vi "Select Display Mode.vi"(8 "error in (no error)":errorcluster, 10 "DisplayMode":T1, 11 "Instruments in":refnum<class "Instruments.lvclass">) -> (0 "error out":errorcluster, 3 "Instruments out":refnum<class "Instruments.lvclass">)   [LabVIEW 2023, in "Instruments.lvlib" / "Instruments.lvclass"]
doc: "Sets the visibility for Waveform, Tables, and Snapshot displays"
uses:
  Library/Instruments.lvclass
  Custom Controls/Display Mode.ctl
  Library/Instruments.lvclass/Instruments.ctl
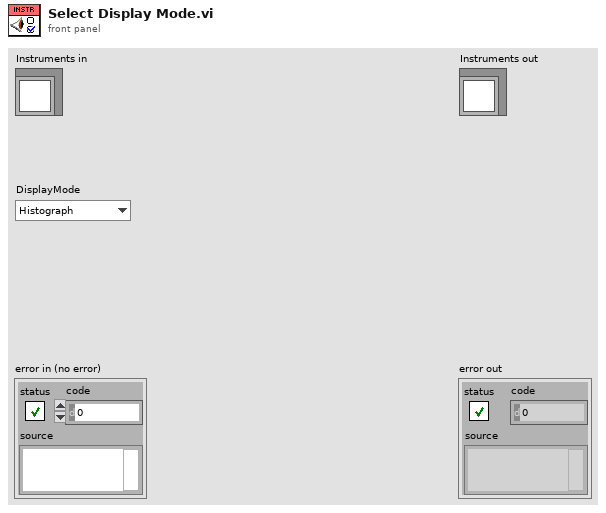
[diagram p1: front panel]
types:
  T1 = typedef "Instruments.lvlib/Instruments.lvclass/Display Mode.ctl" = enum16{"Histograph", "Table", "Snapshot"}
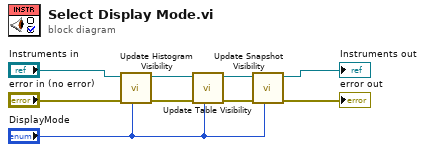
[diagram p0: block diagram]
diagram:
  n1 = call "Update Histogram Visibility.vi"("DisplayMode"="DisplayMode", "error in (no error)"="error in (no error)", "Instruments in"="Instruments in") -> ("error out"=w4:errorcluster, "Instruments out"=w8:refnum<class "Instruments.lvclass">)  [unwired: 7 in]
  n2 = call "Update Table Visibility.vi"("DisplayMode"="DisplayMode", "error in (no error)"=w4, "Instruments in"=w8) -> ("error out"=w3:errorcluster, "Instruments out"=w7:refnum<class "Instruments.lvclass">)  [unwired: 7 in]
  n3 = call "Update Snapshot Visibility.vi"("DisplayMode"="DisplayMode", "error in (no error)"=w3, "Instruments in"=w7) -> ("error out"=→"error out":errorcluster, "Instruments out"=→"Instruments out":refnum<class "Instruments.lvclass">)  [unwired: 7 in]
